vi "GetProjectPath.vi"(1 "File":string) -> (0 "Path":path)   [LabVIEW 2015]
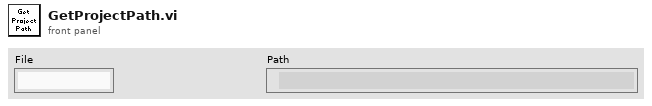
[diagram p1: front panel]
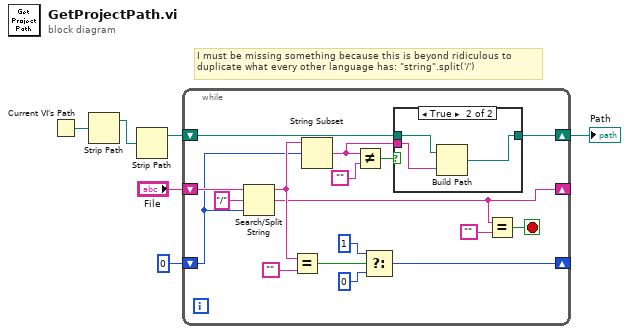
[diagram p0: block diagram]
diagram:
  # "I must be missing something because this is beyond ridiculous to\nduplicate what every other language has: \"string\".split('/')"
  n1 = Current VI's Path() -> (path=w6:path)
  n2 = Strip Path(path=w6) -> (stripped path=w5:path)  [unwired: 1 out]
  n3 = Strip Path(path=w5) -> (stripped path=w2:path)  [unwired: 1 out]
  n4 = while {
    shift-right: [w9] -> _
    shift-left: "File" -> [w22]
    shift-right: [w11] -> _
    shift-left: 0 -> [w19]
    shift-right: [w15] -> w1
    shift-left: w2 -> [w14]
    stop <- w7 stop-if-true
    n5 = Search/Split String(string=w22, search string/char (-)="/", offset (0)=w19) -> (substring before match=w20:string, match + rest of string=w9:string)  [unwired: 1 out]
    n6 = Equal?(x=w20, y="") -> (x = y?=w10:bool)
    n7 = String Subset(string=w20, offset (0)=w19) -> (substring=w16:string)  [unwired: 1 in]
    n8 = Not Equal?(x=w16, y="") -> (x != y?=w18:bool)
    n9 = Select(t=1, s=w10, f=0) -> (s? t:f=w11:i32)
    n10 = case shown="True" w18 {
      tunnel: w16 -> [_ w27]
      tunnel: [w24 w26] -> w15
      tunnel: w14 -> [w24 w25]
      frame False {
      }
      frame True {
        n11 = Build Path(base path=w25, name or relative path=w27) -> (appended path=w26:path)
      }
    }
    n12 = Equal?(x=w9, y="") -> (x = y?=w7:bool)
  }
  "Path" <- w1
